vi "CFTS-Next Data File.vi"(0 "Expt State":T1, 1 "Allow overwrite":bool, 7 "Data Type":T2, 9 "Test only":bool, 11 "error in (no error)":errorcluster) -> (3 "Run #":i16, 4 "Expt State out":T1, 6 "Datafile path":path, 8 "run #":string, 15 "error out":errorcluster)   [LabVIEW 2020]
uses:
  CFTS-Experiment State.ctl
  CFTS-Data Type Enum.ctl
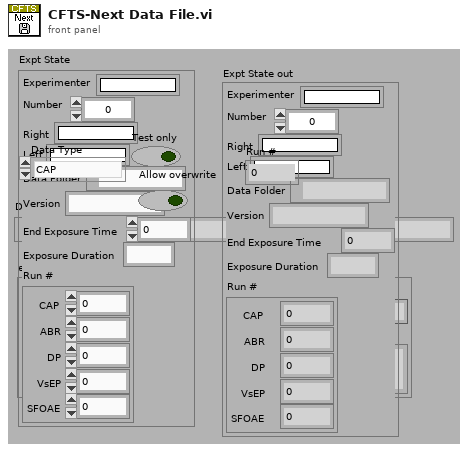
[diagram p1: front panel]
types:
  T1 = typedef "CFTS-Experiment State.ctl" = cluster{"Experimenter":string, "Number":u32, "Right":string, "Left":string, "Data Folder":path, "Version":string, "End Exposure Time":dbl, "Exposure Duration":string, "Run #":cluster{"CAP":i32, "ABR":i32, "DP":i32, "VsEP":i32, "SFOAE":i32}}
  T2 = typedef "CFTS-Data Type Enum.ctl" = enum16{"CAP", "ABR", "DP", "VsEP", "MeasSeq", "SFOAE"}
  T3 = typedef "CFTS-Options.ctl" = cluster{"DP Artifact Rejection":bool, "Monitor vital signs ":bool, "Extension":string}
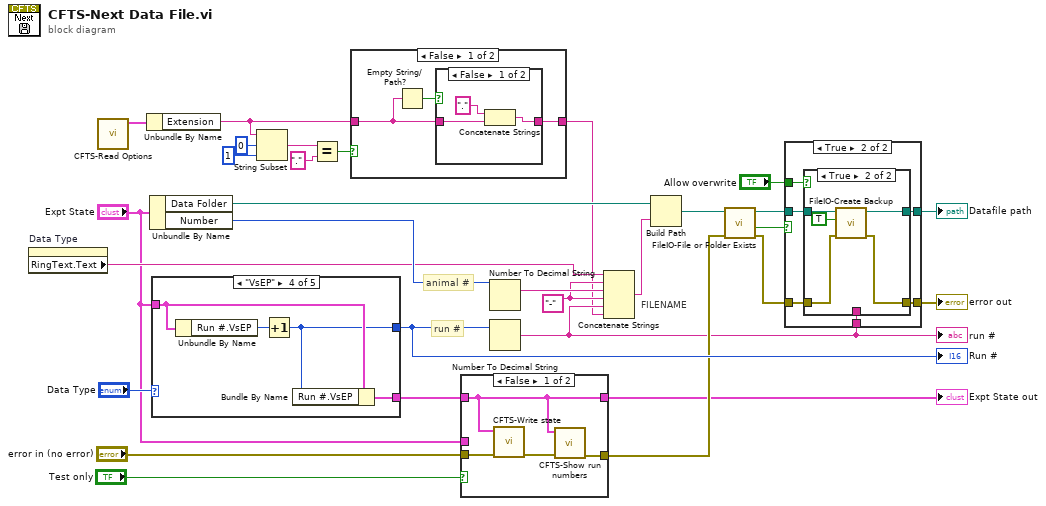
[diagram p0: block diagram]
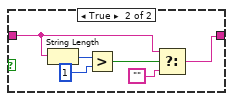
[diagram p3: hidden frame]
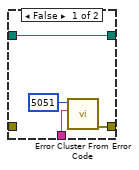
[diagram p6: hidden frame]
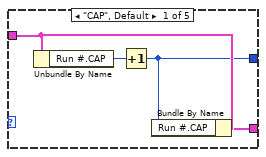
[diagram p7: hidden frame]
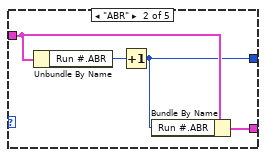
[diagram p8: hidden frame]
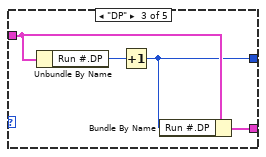
[diagram p9: hidden frame]
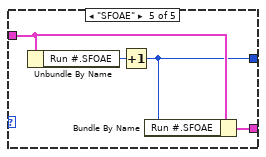
[diagram p10: hidden frame]
diagram:
  w28 = "-"
  # "FILENAME"
  # "animal #"
  # "run #"
  n1 = property on="Data Type" class="Enum (strict)"() -> ("RingText.Text"=w24:string)  [unwired: 2 in, 2 out]
  n2 = call "CFTS-Read Options.vi"() -> ("CFTS Options"=w8:T3)  [unwired: 10 in, 1 out]
  n3 = Unbundle By Name(w8) -> ("Extension"=w2:string)
  n4 = Unbundle By Name("Expt State") -> ("Data Folder"=w27:path, "Number"=w26:u32)
  n5 = case shown="\"VsEP\"" "Data Type" {
    tunnel: "Expt State" -> [w34 w38 w42 w46 w50]
    tunnel: [w32 w36 w40 w44 w48] -> w22
    tunnel: [w31 w35 w39 w43 w47] -> w21
    frame "CAP", Default {
      n6 = Unbundle By Name(w34) -> ("Run #.CAP"=w33:i32)
      n7 = Increment(x=w33) -> (x+1=w31:i32)
      n8 = Bundle By Name(cluster=w34, "Run #.CAP"=w31) -> (w32:T1)
    }
    frame "ABR" {
      n9 = Unbundle By Name(w38) -> ("Run #.ABR"=w37:i32)
      n10 = Increment(x=w37) -> (x+1=w35:i32)
      n11 = Bundle By Name(cluster=w38, "Run #.ABR"=w35) -> (w36:T1)
    }
    frame "DP" {
      n12 = Unbundle By Name(w42) -> ("Run #.DP"=w41:i32)
      n13 = Increment(x=w41) -> (x+1=w39:i32)
      n14 = Bundle By Name(cluster=w42, "Run #.DP"=w39) -> (w40:T1)
    }
    frame "VsEP" {
      n15 = Unbundle By Name(w46) -> ("Run #.VsEP"=w45:i32)
      n16 = Increment(x=w45) -> (x+1=w43:i32)
      n17 = Bundle By Name(cluster=w46, "Run #.VsEP"=w43) -> (w44:T1)
    }
    frame "SFOAE" {
      n18 = Unbundle By Name(w50) -> ("Run #.SFOAE"=w49:i32)
      n19 = Increment(x=w49) -> (x+1=w47:i32)
      n20 = Bundle By Name(cluster=w50, "Run #.SFOAE"=w47) -> (w48:T1)
    }
  }
  "Run #" <- w21
  n21 = String Subset(string=w2, offset (0)=0, length (rest)=1 ("length (rest)")) -> (substring=w5:string)
  n22 = Equal?(x=w5, y=".") -> (x = y?=w3:bool)
  n23 = case shown="False" w3 {
    tunnel: w2 -> [w52 w60]
    tunnel: [w53 w58] -> w1
    frame False {
      n24 = Empty String/Path?(string/path=w52) -> (empty?=w51:bool)
      n25 = case shown="False" w51 {
        tunnel: w52 -> [w56 w57]
        tunnel: [w55 w57] -> w53
        frame False {
          n26 = Concatenate Strings(".", w56) -> (w55:string)
        }
        frame True {
        }
      }
    }
    frame True {
      n27 = String Length(string=w60) -> (length=w63:i32)
      n28 = Greater?(x=w63, y=1) -> (0:w61:bool)
      n29 = Select(t=w60, s=w61, f="") -> (s? t:f=w58:string)
    }
  }
  n30 = case shown="False" "Test only" {
    tunnel: "error in (no error)" -> [w67 w69]
    tunnel: w22 -> [w64 _]
    tunnel: [w65 w69] -> w19
    tunnel: [w64 w68] -> w13
    tunnel: "Expt State" -> [_ w68]
    frame False {
      n31 = call "CFTS-Write state.vi"("error in (no error)"=w67, "Experiment info"=w64) -> ("error out"=w66:errorcluster)  [unwired: 9 in]
      n32 = call "CFTS-Show run numbers.vi"("error in (no error)"=w66, "Expt State"=w64) -> ("error out"=w65:errorcluster)  [unwired: 9 in]
    }
    frame True {
    }
  }
  "Expt State out" <- w13
  n33 = Number To Decimal String(number=w26) -> (decimal integer string=w30:string)  [unwired: 1 in]
  n34 = Number To Decimal String(number=w21) -> (decimal integer string=w15:string)  [unwired: 1 in]
  "run #" <- w15
  n35 = Concatenate Strings(w24, w28, w30, w28, w15, w1) -> (w29:string)
  n36 = Build Path(base path=w27, name or relative path=w29) -> (appended path=w20:path)
  n37 = call "FileIO-File or Folder Exists.vi"("error in (no error)"=w19, "path"=w20) -> ("error out"=w17:errorcluster, "Exists?"=w18:bool, "dup path"=w11:path)  [unwired: 6 in, 1 out]
  n38 = case shown="True" w18 {
    tunnel: w17 -> [w71 w72]
    tunnel: [w71 w77] -> w16
    tunnel: w15 -> [_ w76]
    tunnel: w11 -> [w70 w74]
    tunnel: [w70 w73] -> w10
    tunnel: "Allow overwrite" -> [_ w75]
    frame False {
    }
    frame True {
      n39 = case shown="True" w75 {
        tunnel: [w81 w83] -> w77
        tunnel: w76 -> [w79 _]
        tunnel: w74 -> [w78 w86]
        tunnel: [w78 w85] -> w73
        tunnel: w72 -> [_ w84]
        frame False {
          n40 = call <vilib>:"Error Cluster From Error Code.vi"("error message (\"\")"=w79, "error code (0)"=5051) -> ("error out"=w81:errorcluster)  [unwired: 7 in]
        }
        frame True {
          n41 = call "FileIO-Create Backup.vi"("error in (no error)"=w84, "Delete tag"=TRUE, "Path"=w86) -> ("error out"=w83:errorcluster, "Path (thru)"=w85:path)  [unwired: 5 in, 2 out]
        }
      }
    }
  }
  "error out" <- w16
  "Datafile path" <- w10
